vi "11- Peak detector (SubVI).vi"(11 "Input peak level":dbl=10.0) -> (1 "Number of peaks":i32, 2 "Indexes of peaks":i32[](array[numeric]), 3 "Array":dbl[](array[numeric]))   [LabVIEW 2019]
panel:
  # "PEAK DETECTOR SUBVI"
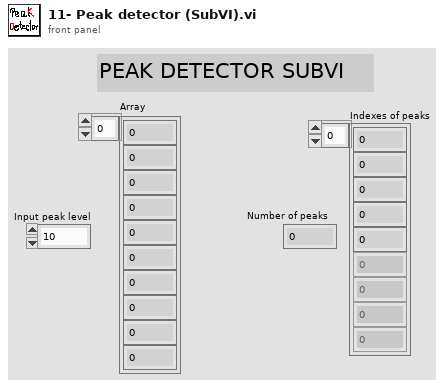
[diagram p1: front panel]
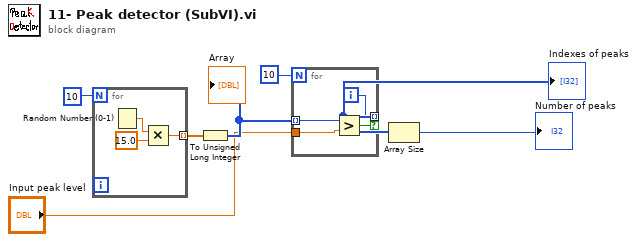
[diagram p0: block diagram]
diagram:
  n1 = for {
    N: 10 -> [_]
    tunnel: [w8] -> w4 mode=indexing
    n2 = Random Number (0-1)() -> (number: 0 to 1=w10:dbl)
    n3 = Multiply(x=w10, y=15.0 ("x")) -> (x*y=w8:dbl)
  }
  n4 = To Unsigned Long Integer(number=w4) -> (unsigned 32bit integer=w5:u32[])
  "Array" <- w5
  n5 = for {
    N: 10 -> [_]
    tunnel: w5 -> [w14] mode=indexing
    tunnel: "Input peak level" -> [w13]
    tunnel: [w12] -> w6 mode=indexing if=w11
    i -> [w12]
    n6 = Greater?(x=w14, y=w13) -> (0:w11:bool)
  }
  "Indexes of peaks" <- w6
  n7 = Array Size(array=w6) -> (size(s)=→"Number of peaks":i32)
